vi "Get Top Most Crates.vi"(1 "Cargo":T1) -> (0 "Top Most Crates":string)   [LabVIEW 2020, in "AoC 2022.lvlib"]
uses:
  AoC 2022.lvlib
  Cargo.ctl
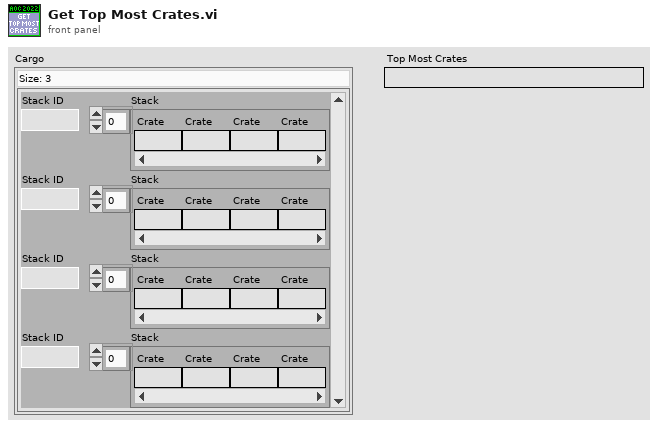
[diagram p1: front panel]
types:
  T1 = typedef "AoC 2022.lvlib/Cargo.ctl" = map{i32, string[]}
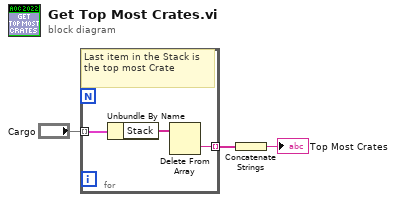
[diagram p0: block diagram]
diagram:
  n1 = for {
    tunnel: "Cargo" -> [w6] mode=indexing
    tunnel: [w4] -> w2 mode=indexing
    # "Last item in the Stack is the top most Crate"
    n2 = Unbundle By Name(w6) -> ("Stack"=w5:string[])
    n3 = Delete From Array(array=w5) -> (deleted portion=w4:string)  [unwired: 2 in, 1 out]
  }
  n4 = Concatenate Strings(w2) -> (→"Top Most Crates":string)
